vi "magspec stitcher get pixel to insert interp image.vi"(9 "Delta":dbl, 10 "min X of all":dbl, 11 "min X of current":dbl) -> (2 "x pixel double prec":dbl, 3 "X pixel to insert into":i32)   [LabVIEW 2020]
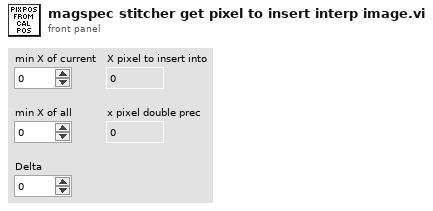
[diagram p1: front panel]
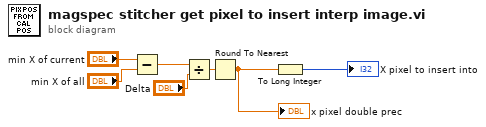
[diagram p0: block diagram]
diagram:
  n1 = Subtract(x="min X of current", y="min X of all") -> (x-y=w1:dbl)
  n2 = Divide(x=w1, y="Delta") -> (x/y=w3:dbl)
  n3 = Round To Nearest(number=w3) -> (nearest integer value=w6:dbl)
  "x pixel double prec" <- w6
  n4 = To Long Integer(number=w6) -> (32bit integer=→"X pixel to insert into":i32)
